vi "DAQ_Accelerometer_ch.vi"(9 "channel":T1) -> ()   [LabVIEW 2020]
uses:
  <extravilib>/ChannelInstances/Tag-bool/))Channel.ctl
  <extravilib>/ChannelInstances/Tag-bool/Read With Abort.vi
  <extravilib>/ChannelInstances/Tag-bool/EndpointRead.vi
  <extravilib>/ChannelInstances/Tag-bool.lvlib
panel:
  out "Waveform Graph":dynamicdata(graph)
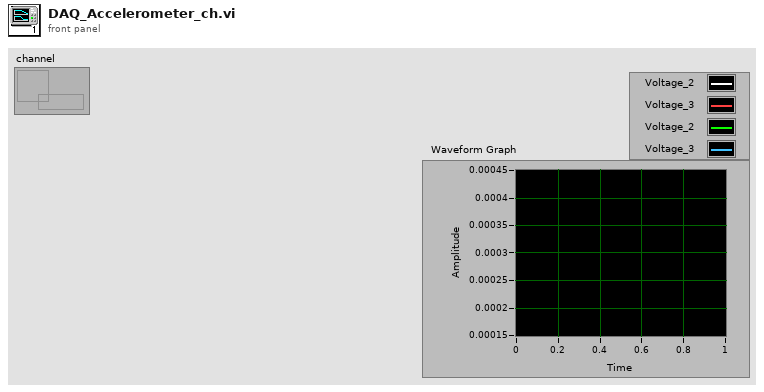
[diagram p1: front panel]
types:
  T1 = typedef "Tag-bool.lvlib/))Channel.ctl" = refnum<queue>
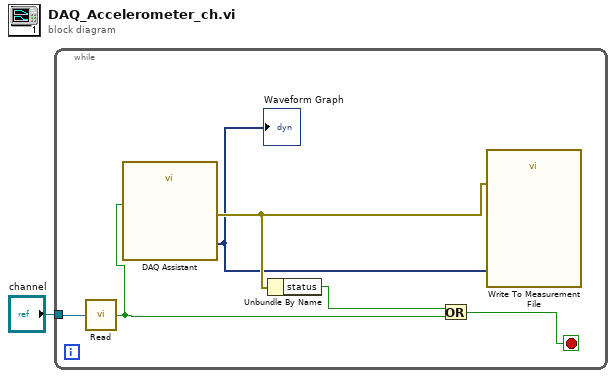
[diagram p0: block diagram]
diagram:
  n1 = while {
    tunnel: "channel" -> [w2]
    stop <- w5 stop-if-true
    n2 = call <extravilib>:"Read.vi"("channel"=w2) -> ("element"=w3:bool)  [unwired: 1 in, 1 out]
    n3 = call "DAQ Assistant"("stop (T)"=w3) -> ("data"=w4:dynamicdata, "error out"=w6:errorcluster)  [unwired: 16 in, 1 out]
    "Waveform Graph" <- w4
    n4 = Unbundle By Name(w6) -> ("status"=w7:bool)
    n5 = Or(x=w7, y=w3) -> (x .or. y?=w5:bool)
    n6 = call "Write To Measurement File"("Signals"=w4, "error in (no error)"=w6) -> ()  [unwired: 15 in, 3 out]
  }
